vi "RT Main.vi"() -> ()   [LabVIEW 2015]
uses:
  <vilib>/robotics/Navigation/shared/WorldMap/DirectedGraphWorldMap/NI_Robotics_DirectedGraphWorldMap.lvclass
  NI-ARC 2017/NI ARC 2016/Types/Status.ctl
  Types/Mode.ctl
  <vilib>/myRIO/Instrument Drivers/Onboard IO/DIO/typedefs/DIO Reference.ctl
  <vilib>/myRIO/Common/Instrument Driver Framework/Utilities/typedefs/myRIO Generic Hardware Reference.ctl
  <vilib>/myRIO/Common/Instrument Driver Framework/Utilities/typedefs/Hardware Version Enum.ctl
  <vilib>/myRIO/Common/Instrument Driver Framework/Utilities/typedefs/myRIO v1.0 Reference.ctl
  <vilib>/myRIO/Common/Instrument Driver Framework/Utilities/typedefs/Generic FPGA Reference.ctl
  <vilib>/myRIO/Common/Instrument Driver Framework/myRIO v1.0/DIO/typedefs/DIO Channels List.ctl
  <vilib>/myRIO/Common/Instrument Driver Framework/myRIO v1.0/DIO/typedefs/DIO Channels Enum.ctl
  <vilib>/userdefined/High Color/nirio_resource_hc.ctl
  <vilib>/myRIO/Common/Instrument Driver Framework/Utilities/vis/Is FPGA Ref Available.vi
  <vilib>/myRIO/Common/Instrument Driver Framework/myRIO v1.0/DIO/vis/myRIO v1.1 Open DIO.vi
  <vilib>/myRIO/Instrument Drivers/Onboard IO/DIO/vis/Read.vi
  <vilib>/myRIO/Instrument Drivers/Onboard IO/DIO/vis/Write.vi
  <vilib>/myRIO/Common/Instrument Driver Framework/Utilities/vis/Validate Channels.vi
  <vilib>/myRIO/Common/Instrument Driver Framework/myRIO v1.0/DIO/vis/myRIO v1.0 Reserve DIO.vi
  <vilib>/myRIO/Common/Instrument Driver Framework/myRIO v1.0/Resource Manager/vis/myRIO v1.0 Reserve Channel List.vi
  <vilib>/myRIO/Common/Instrument Driver Framework/myRIO v1.0/DIO/vis/myRIO v1.0 Build MUX Configuration DIO.vi
  <vilib>/myRIO/Common/Instrument Driver Framework/myRIO v1.0/Resource Manager/vis/myRIO v1.0 Reserve Channel.vi
  <vilib>/myRIO/Common/Instrument Driver Framework/myRIO v1.0/Resource Manager/vis/myRIO v1.0 Unreserve Channel.vi
  <vilib>/myRIO/Common/Instrument Driver Framework/myRIO v1.0/Resource Manager/vis/myRIO v1.0 Create Configuration List.vi
  <vilib>/myRIO/Common/Instrument Driver Framework/myRIO v1.0/Resource Manager/vis/myRIO v1.0 Build Mutex Name.vi
  <vilib>/Utility/tcp.llb/UDP Multicast Read-Only Open.vi
  <vilib>/FPGAPlugInAG/myRIO-1900/niLvFpga_Open_myRIO-1900.vi
  <vilib>/rvi/interface/common/dynamic/niFpgaDynamicAddResources.vi
  <vilib>/myRIO/Common/Instrument Driver Framework/Utilities/vis/FPGA Ref Manager.vi
  <vilib>/Utility/error.llb/Error Cluster From Error Code.vi
  <vilib>/myRIO/Common/Instrument Driver Framework/Utilities/vis/Ref Counter.vi
  <vilib>/Utility/VariantDataType/GetNumericInfo.vi
  <vilib>/myRIO/Common/Instrument Driver Framework/myRIO v1.0/myRIO v1.1 Open.vi
  <vilib>/myRIO/Common/Instrument Driver Framework/Utilities/vis/IO Manager.vi
  <vilib>/myRIO/Common/Instrument Driver Framework/Utilities/vis/Configuration Manager.vi
  <vilib>/myRIO/Common/Instrument Driver Framework/myRIO v1.0/Resource Manager/vis/myRIO v1.0 Configure IO.vi
  <vilib>/myRIO/Common/Instrument Driver Framework/myRIO v1.0/myRIO v1.0 Close.vi
  <vilib>/myRIO/Common/Instrument Driver Framework/myRIO v1.0/DIO/vis/myRIO v1.0 Read DIO.vi
  <vilib>/myRIO/Common/Instrument Driver Framework/myRIO v1.0/DIO/vis/myRIO v1.0 Write DIO.vi
  <vilib>/FPGAPlugInAG/Dynamic/niLvFpga_Close_Dynamic.vi
  <vilib>/rvi/interface/nirviOpenFPGA/nirviOpenFPGA.xnode
  FPGA Bitfiles/NIARC2017_FPGATarget_FPGAMainDefault_FCosad5cmWo.lvbitx
  <vilib>/myRIO/Express VI/Onboard IO/DI/DI Express VI.xnode
  <vilib>/myRIO/Instrument Drivers/Onboard IO/DIO/vis/myRIO DIO Open.xnode
  <vilib>/myRIO/Express VI/Onboard IO/DO/DO Express VI.xnode
  <vilib>/rvi/interface/nirviCloseFPGA/nirviCloseFPGA.xnode
  <instrlib>/Hokuyo URG Series/HAIOL/Hokuyo URG Series.lvclass
  <vilib>/myRIO/Instrument Drivers/Utilities/Utilities.lvlib
  <instrlib>/Hokuyo URG Series/HAIOL/VISA/Hokuyo URG Series VISA.lvclass
  <vilib>/myRIO/Instrument Drivers/Onboard IO/DIO/DIO.lvlib
panel:
  in  "LidarDetection":bool
  out "x*y":dbl
  out "Next":T1
  out "wifiClosures":bool[](array[boolean])
  in  "MovingRobot":bool
  in  "Mode":T2
  in  "Status":T3
  out "Closures":bool[](array[boolean])
  out "closeLidar":cluster{dbl, dbl}[](array[cluster])
  out "Returning":bool=TRUE
  out "Last":string
  out "Wifi String":string
  out "error out":errorcluster
  out "Path":cluster{"name":string, "coordinates":dbl[]}[](array[cluster])
  out "Vertical Closures":bool[](array[boolean])
  in  "6":bool
  in  "5":bool
  in  "8":bool
  in  "7":bool
  in  "4":bool
  in  "3":bool
  in  "2":bool
  in  "1":bool
  out "No Valid Path":bool
  out "Horizontal Closures":bool[](array[boolean])
  in  "I":bool
  in  "H":bool
  in  "G":bool
  in  "F":bool
  in  "E":bool
  in  "D":bool
  in  "C":bool
  in  "B":bool
  in  "A":bool
  out "MapOut":refnum<data-value>
  out "Zones":T4(array[cluster])
  out "Obstacles":T4(array[cluster])
  out "Instruction":u32
  out "Start":T5
  in  "Finished":bool
  out "currentPath":T6
  out "Path":T7(array[cluster])=[{"pathSegment"={"Point 1"={"X"=250.0, "Y"=250.0}, "Point 2"={"X"=500.0, "Y"=250.0}}, "targetAngle"=0.0, "Speed"=1.0}, {"pathSegment"={"Point 1"={"X"=500.0, "Y"=250.0}, "Point 2"={"X"=300.0, "Y"=1500.0}}, "targetAngle"=90.0, "Speed"=1.0}, {"pathSegment"={"Point 1"={"X"=300.0, "Y"=1500.0}, "Point 2"={"X"=500.0, "Y"=3700.0}}, "targetAngle"=90.0, "Speed"=1.0}, {"pathSegment"={"Point 1"={"X"=500.0, "Y"=3700.0}, "Point 2"={"X"=3000.0, "Y"=3700.0}}, "targetAngle"=0.0, "Speed"=1.0}]
  out "plotPoints":cluster{dbl, dbl}[](array[cluster])
  out "Map":T8(plugin-control)
  out "lidarObstacles":T4(array[cluster])
  out "verticalCourse":cluster{"X":sgl, "Y":sgl}[](array[cluster])=[{"X"=-400.0, "Y"=600.0}, {"X"=-200.0, "Y"=600.0}, {"X"=0.0, "Y"=600.0}, {"X"=200.0, "Y"=600.0}, {"X"=400.0, "Y"=600.0}]
  out "hoizontalCourse":cluster{"X":sgl, "Y":sgl}[](array[cluster])=[{"X"=-400.0, "Y"=600.0}, {"X"=-200.0, "Y"=600.0}, {"X"=0.0, "Y"=600.0}, {"X"=200.0, "Y"=600.0}, {"X"=400.0, "Y"=600.0}]
  out "robotPosition":T5
  in  "Enable Motors":bool
  in  "Stop":bool
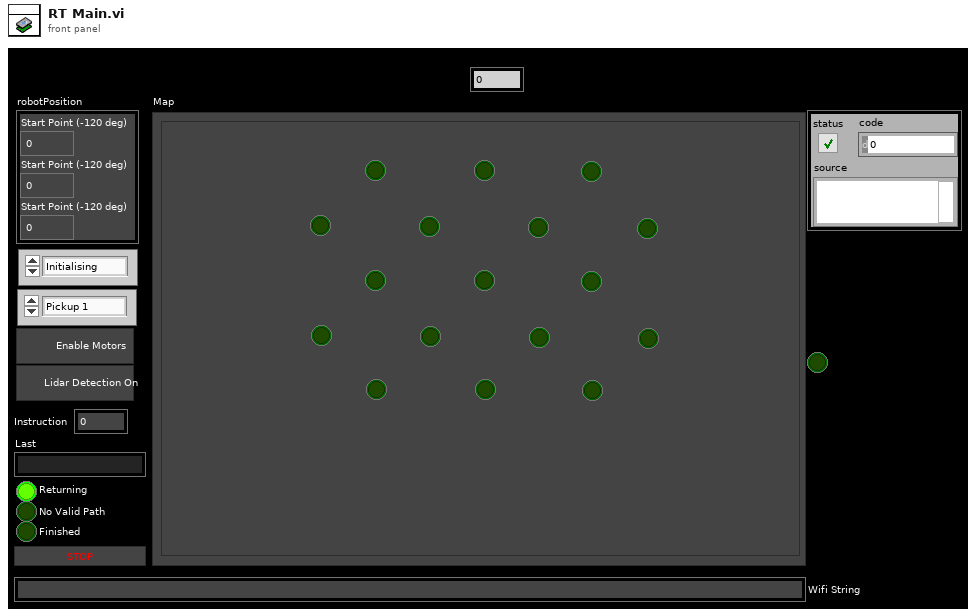
[diagram p1: front panel]
types:
  T1 = cluster{cluster{cluster{"Numeric":dbl, "Numeric":dbl}, cluster{"Numeric":dbl, "Numeric":dbl}}, "Ramp (V/s)":dbl, "Ramp (V/s)":dbl, bool}
  T2 = typedef "Mode.ctl" = enum16{"Pickup 1", "Pickup 2", "Moving Robot"}
  T3 = typedef "Status.ctl" = enum16{"Initialising", "Waiting", "Go"}
  T4 = cluster{"Point 1":cluster{"X":sgl, "Y":sgl}, "Point 2":cluster{"X":sgl, "Y":sgl}}[]
  T5 = cluster{"Start Point (-120 deg)":dbl, "Start Point (-120 deg)":dbl, "Start Point (-120 deg)":dbl}
  T6 = cluster{"pathSegment":cluster{"Point 1":cluster{"X":sgl, "Y":sgl}, "Point 2":cluster{"X":sgl, "Y":sgl}}, "targetAngle":dbl, "Speed":dbl}
  T7 = cluster{"pathSegment":cluster{"Point 1":cluster{"X":sgl, "Y":sgl}, "Point 2":cluster{"X":sgl, "Y":sgl}}, "targetAngle":dbl, "Speed":dbl}[]
  T8 = typedef "IMAQ Image.ctl" = refnum<image>
  T9 = typedef "DIO.lvlib/DIO Reference.ctl" = cluster{"myRIO Reference":T10, "DIO Channels List":T14}
  T10 = typedef "myRIO Generic Hardware Reference.ctl" = cluster{"myRIO Model":T11, "myRIO Hardware Reference":T12}
  T11 = typedef "Hardware Version Enum.ctl" = enum16{"Unknown", "myRIO-1900", "myRIO-1950", "roboRIO"}
  T12 = typedef "myRIO v1.0 Reference.ctl" = cluster{"Generic FPGA Reference":T13, "Allow multiple opens":bool}
  T13 = typedef "Generic FPGA Reference.ctl" = refnum<k20>
  T14 = typedef "DIO Channels List.ctl" = T15[]
  T15 = typedef "DIO Channels Enum.ctl" = enum16{"Not Connected", "C/DIO0", "C/DIO1", "C/DIO2", "C/DIO3", "C/DIO4", "C/DIO5", "C/DIO6", "C/DIO7", "A/DIO0", "A/DIO1", "A/DIO2", "A/DIO3", "A/DIO4", "A/DIO5", "A/DIO6", "A/DIO7", "A/DIO8", "A/DIO9", "A/DIO10", "A/DIO11", "A/DIO12", "A/DIO13", "A/DIO14", "A/DIO15", "B/DIO0", "B/DIO1", "B/DIO2", "B/DIO3", "B/DIO4", "B/DIO5", "B/DIO6", "B/DIO7", "B/DIO8", "B/DIO9", "B/DIO10", "B/DIO11", "B/DIO12", "B/DIO13", "B/DIO14", "B/DIO15", "LED0", "LED1", "LED2", "LED3", "Button0", "DIO/DIO0", "DIO/DIO1", "DIO/DIO2", "DIO/DIO3", "DIO/DIO4", "DIO/DIO5", "DIO/DIO6", "DIO/DIO7", "DIO/DIO8", "DIO/DIO9", "SPI/CS0", "SPI/CS1", "SPI/CS2", "SPI/CS3", "LED RADIO (Green)", "LED RADIO (Red)", "LED COMM (Green)", "LED COMM (Red)", "LED MODE (Green)", "LED MODE (Red)"}
  T16 = typedef "nirio_resource_hc.ctl" = tag
  T17 = cluster{cluster{cluster{"Numeric":dbl, "Numeric":dbl}, cluster{"Numeric":dbl, "Numeric":dbl}}, "Ramp (V/s)":dbl, "Ramp (V/s)":dbl}
  T18 = cluster{"Point 1":cluster{"X":sgl, "Y":sgl}, "Point 2":cluster{"X":sgl, "Y":sgl}}
  T19 = cluster{"x-Error":dbl, "y-Error":dbl, "Angle-Error (deg)":dbl}
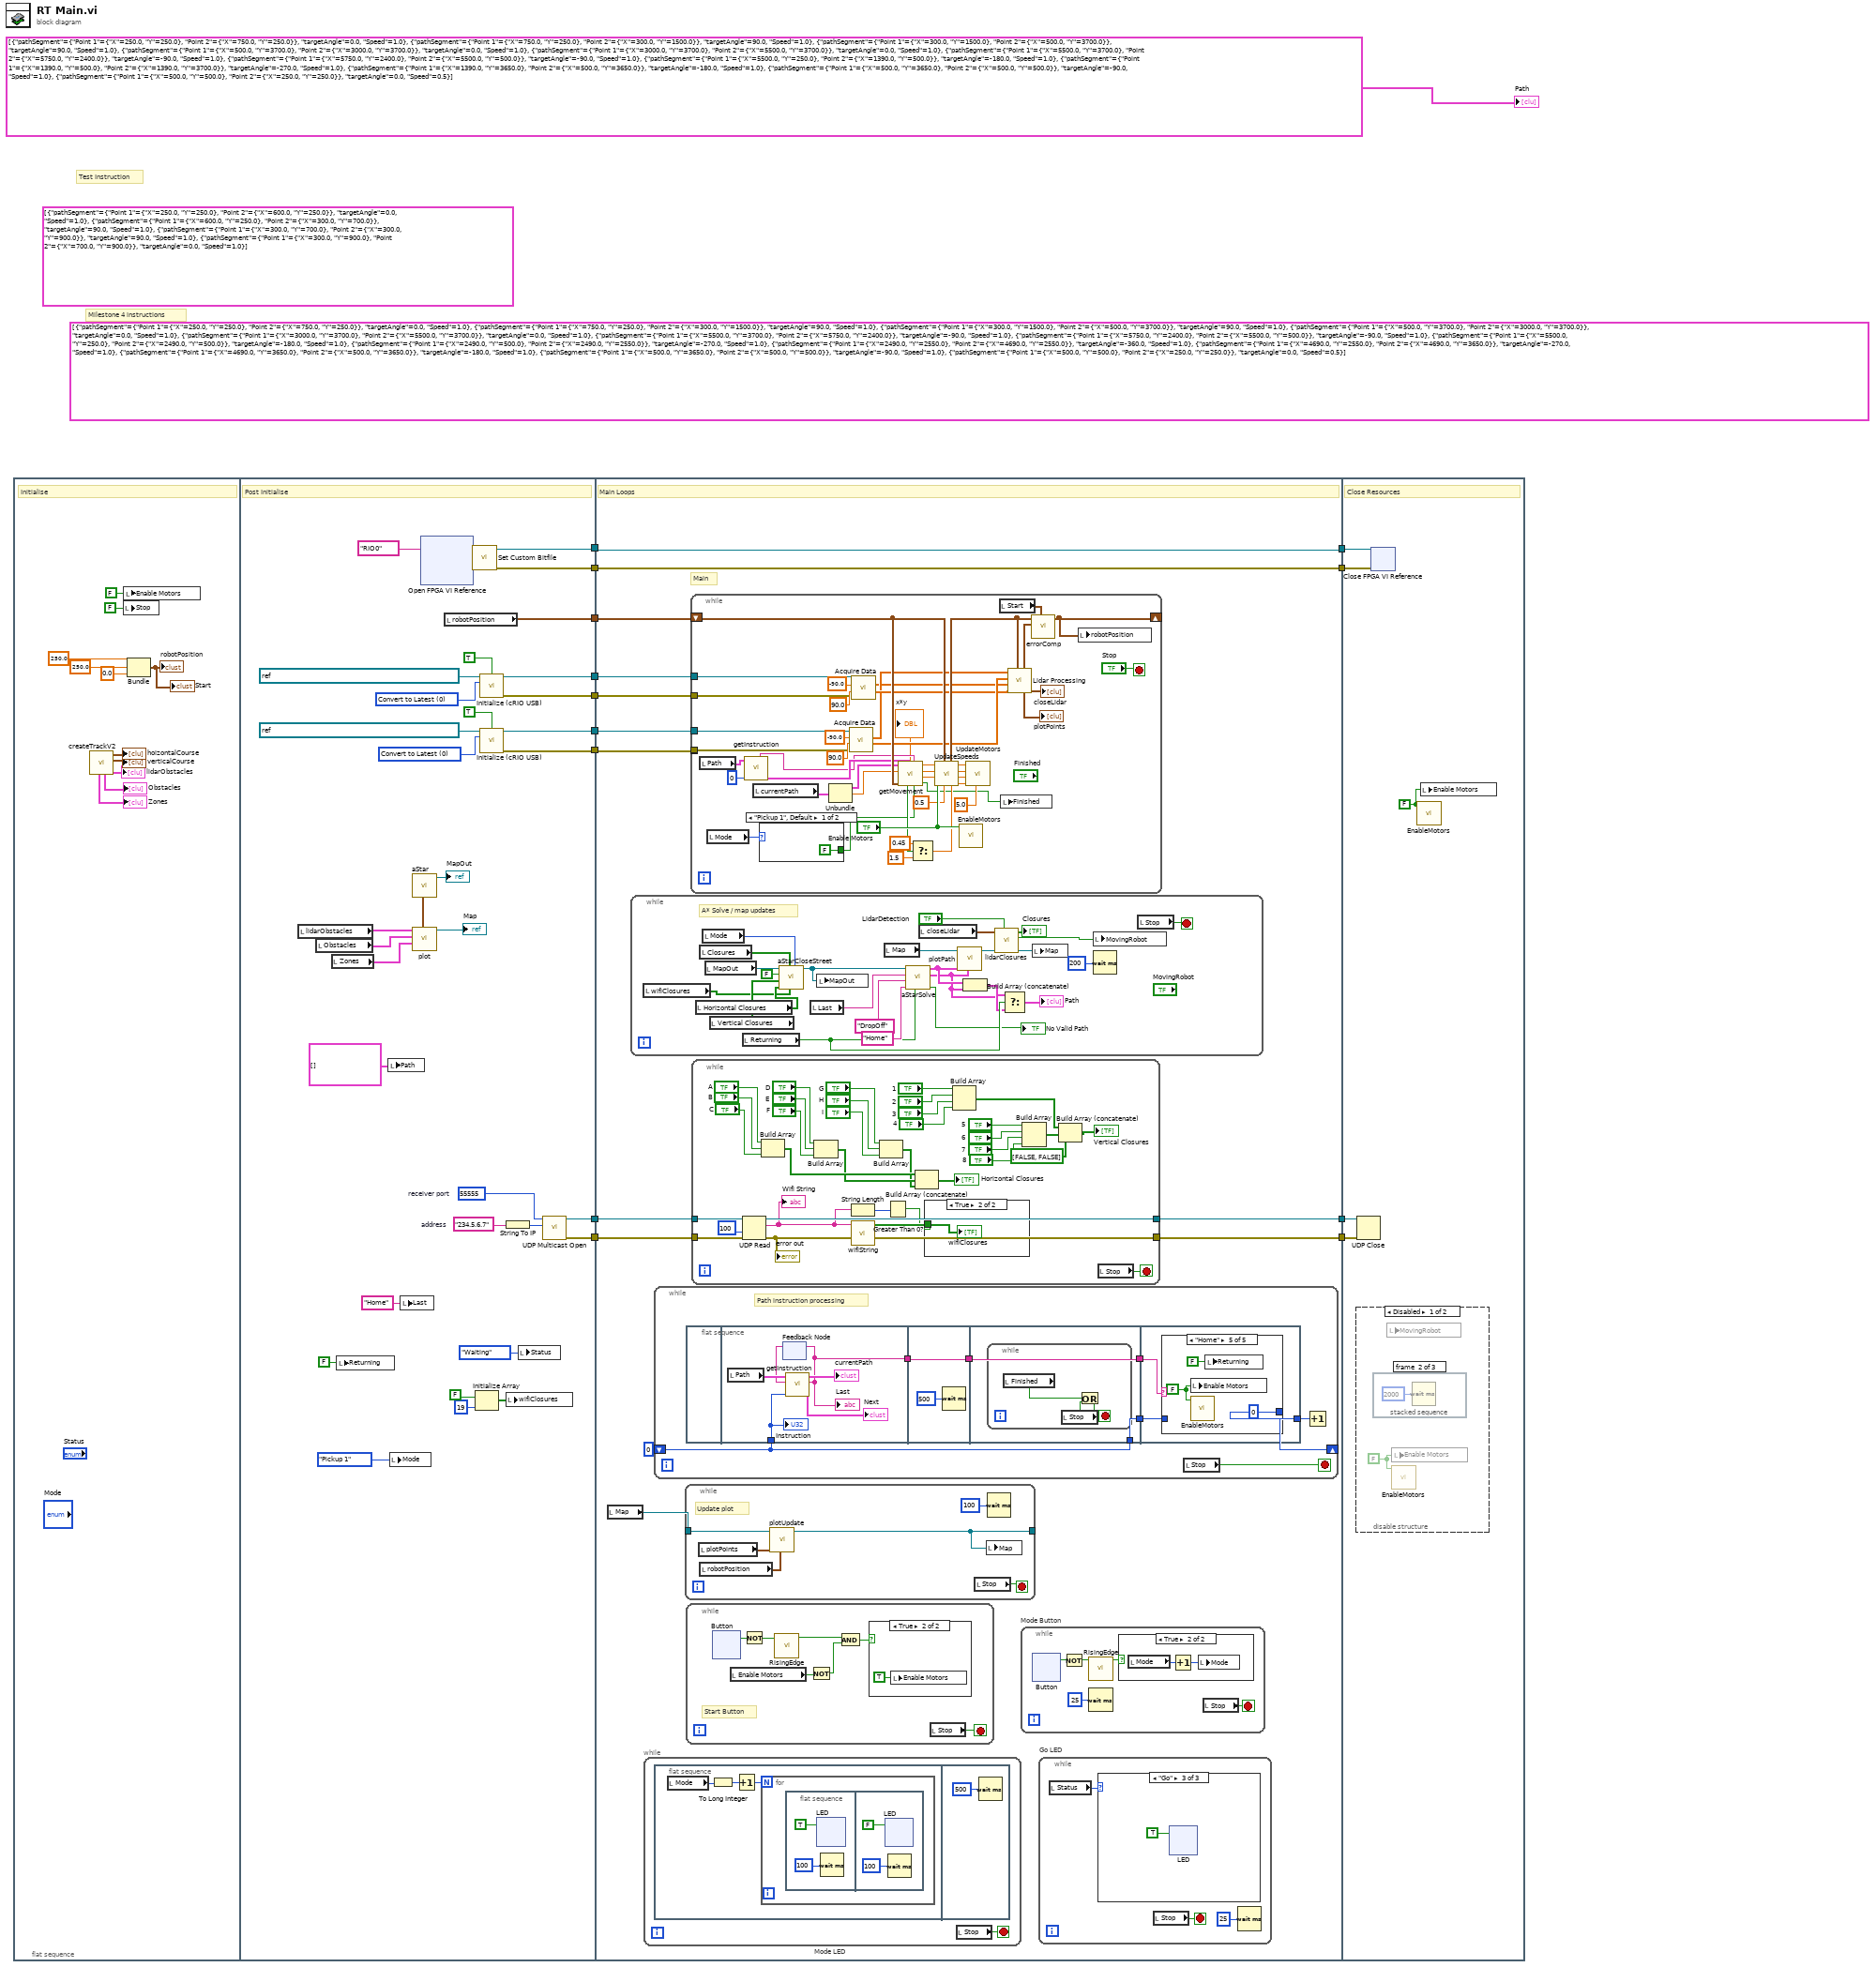
[diagram p0: block diagram]
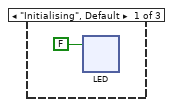
[diagram p3: hidden frame]
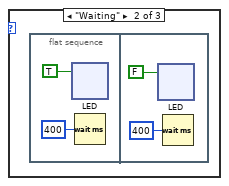
[diagram p4: hidden frame]
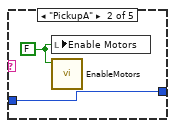
[diagram p8: hidden frame]
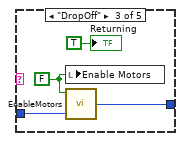
[diagram p9: hidden frame]
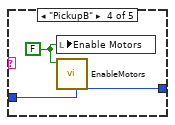
[diagram p10: hidden frame]
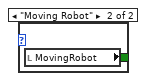
[diagram p11: hidden frame]
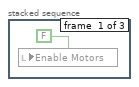
[diagram p12: hidden frame]
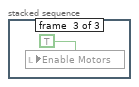
[diagram p13: hidden frame]
diagram:
  (unwired) T7 [{"pathSegment"={"Point 1"={"X"=250.0, "Y"=250.0}, "Point 2"={"X"=600.0, "Y"=250.0}}, "targetAngle"=0.0, "Speed"=1.0}, {"pathSegment"={"Point 1"={"X"=600.0, "Y"=250.0}, "Point 2"={"X"=300.0, "Y"=700.0}}, "targetAngle"=90.0, "Speed"=1.0}, {"pathSegment"={"Point 1"={"X"=300.0, "Y"=700.0}, "Point 2"={"X"=300.0, "Y"=900.0}}, "targetAngle"=90.0, "Speed"=1.0}, {"pathSegment"={"Point 1"={"X"=300.0, "Y"=900.0}, "Point 2"={"X"=700.0, "Y"=900.0}}, "targetAngle"=0.0, "Speed"=1.0}]
  (unwired) T7 [{"pathSegment"={"Point 1"={"X"=250.0, "Y"=250.0}, "Point 2"={"X"=750.0, "Y"=250.0}}, "targetAngle"=0.0, "Speed"=1.0}, {"pathSegment"={"Point 1"={"X"=750.0, "Y"=250.0}, "Point 2"={"X"=300.0, "Y"=1500.0}}, "targetAngle"=90.0, "Speed"=1.0}, {"pathSegment"={"Point 1"={"X"=300.0, "Y"=1500.0}, "Point 2"={"X"=500.0, "Y"=3700.0}}, "targetAngle"=90.0, "Speed"=1.0}, {"pathSegment"={"Point 1"={"X"=500.0, "Y"=3700.0}, "Point 2"={"X"=3000.0, "Y"=3700.0}}, "targetAngle"=0.0, "Speed"=1.0}, {"pathSegment"={"Point 1"={"X"=3000.0, "Y"=3700.0}, "Point 2"={"X"=5500.0, "Y"=3700.0}}, "targetAngle"=0.0, "Speed"=1.0}, {"pathSegment"={"Point 1"={"X"=5500.0, "Y"=3700.0}, "Point 2"={"X"=5750.0, "Y"=2400.0}}, "targetAngle"=-90.0, "Speed"=1.0}, {"pathSegment"={"Point 1"={"X"=5750.0, "Y"=2400.0}, "Point 2"={"X"=5500.0, "Y"=500.0}}, "targetAngle"=-90.0, "Speed"=1.0}, {"pathSegment"={"Point 1"={"X"=5500.0, "Y"=250.0}, "Point 2"={"X"=2490.0, "Y"=500.0}}, "targetAngle"=-180.0, "Speed"=1.0}, {"pathSegment"={"Point 1"={"X"=2490.0, "Y"=500.0}, "Point 2"={"X"=2490.0, "Y"=2550.0}}, "targetAngle"=-270.0, "Speed"=1.0}, {"pathSegment"={"Point 1"={"X"=2490.0, "Y"=2550.0}, "Point 2"={"X"=4690.0, "Y"=2550.0}}, "targetAngle"=-360.0, "Speed"=1.0}, {"pathSegment"={"Point 1"={"X"=4690.0, "Y"=2550.0}, "Point 2"={"X"=4690.0, "Y"=3650.0}}, "targetAngle"=-270.0, "Speed"=1.0}, {"pathSegment"={"Point 1"={"X"=4690.0, "Y"=3650.0}, "Point 2"={"X"=500.0, "Y"=3650.0}}, "targetAngle"=-180.0, "Speed"=1.0}, {"pathSegment"={"Point 1"={"X"=500.0, "Y"=3650.0}, "Point 2"={"X"=500.0, "Y"=500.0}}, "targetAngle"=-90.0, "Speed"=1.0}, {"pathSegment"={"Point 1"={"X"=500.0, "Y"=500.0}, "Point 2"={"X"=250.0, "Y"=250.0}}, "targetAngle"=0.0, "Speed"=0.5}]
  # "Milestone 4 instructions"
  # "Test Instruction"
  n1 = flat-sequence {
    tunnel: [w57] -> w14
    tunnel: [w56] -> w13
    tunnel: [w53] -> w12
    tunnel: [w52] -> w11
    tunnel: [w51] -> w8
    tunnel: [w42] -> w6
    tunnel: [w41] -> w5
    tunnel: [w35] -> w4
    tunnel: [w34] -> w3
    tunnel: w14 -> [w71]
    tunnel: w13 -> [w70]
    tunnel: w12 -> [w73]
    tunnel: w11 -> [w72]
    tunnel: [w71] -> w10
    tunnel: [w70] -> w9
    tunnel: w8 -> [w69]
    tunnel: w6 -> [w66]
    tunnel: w5 -> [w65]
    tunnel: w4 -> [w64]
    tunnel: w3 -> [w63]
    tunnel: [w62] -> w2
    tunnel: [w61] -> w1
    tunnel: w10 -> [w540]
    tunnel: w9 -> [w539]
    tunnel: w2 -> [w537]
    tunnel: w1 -> [w536]
    frame #0 {
      # "Initialise"
      n2 = call "createTrackV2.vi"() -> ("lidarObstacles"=→"lidarObstacles":T4, "verticalCourse"=→"verticalCourse":cluster{"X":sgl, "Y":sgl}[], "hoizontalCourse"=→"hoizontalCourse":cluster{"X":sgl, "Y":sgl}[], "obstacles"=→"Obstacles":T4, "Zones"=→"Zones":T4)  [unwired: 7 in]
      n3 = local write "Stop"(FALSE ("Stop")) -> ()
      n4 = local write "Enable Motors"(FALSE ("Enable Motors")) -> ()
      n5 = Bundle("Start Point (-120 deg)"=250.0, "Start Point (-120 deg)"=250.0, "Start Point (-120 deg)"=0.0) -> (→"robotPosition" →"Start":T5)  [unwired: 1 in]
    }
    frame #1 {
      w37 = u16 55555  # receiver port
      w38 = "234.5.6.7"  # address
      w44 = u32 0 items=["Convert to Latest", "SCIP 1.1", "SCIP 2.0"] ("Protocol (2: SCIP 2.0)")
      w54 = u32 0 items=["Convert to Latest", "SCIP 1.1", "SCIP 2.0"] ("Protocol (2: SCIP 2.0)")
      # "Post Initialise"
      n6 = local read "lidarObstacles"() -> (w50:T4)
      n7 = local read "Obstacles"() -> (w48:T4)
      n8 = local read "Zones"() -> (w47:T4)
      n9 = local write "Returning"(FALSE ("Returning")) -> ()
      n10 = local write "Path"(cluster{"name":string, "coordinates":dbl[]}[] [] ("Path")) -> ()
      n11 = local write "Mode"(Mode."Pickup 1" ("Mode")) -> ()
      n12 = local write "Last"("Home" ("Last")) -> ()
      n13 = call "aStar.vi"() -> ("MapOut"=→"MapOut":refnum<data-value>, "wayPoints"=w40:cluster{"Numeric":dbl, "Numeric":dbl}[])  [unwired: 10 in]
      n14 = call "plot.vi"("wayPoints"=w40, "Zones"=w47, "Obstacles"=w48, "Lidar"=w50) -> ("Image"=→"Map":T8)  [unwired: 7 in]
      n15 = xnode "Open FPGA VI Reference"("resource name"=tag "RIO0") -> ("FPGA VI Reference Out"=w58:refnum<k20>, "error out"=w59:errorcluster)  [unwired: 1 in]
      n16 = local read "robotPosition"() -> (w51:T5)
      n17 = call <vilib>:"Set Custom Bitfile.vi"("error in (no error)"=w59, "Custom FPGA Reference In"=w58) -> ("error out"=w56:errorcluster, "Custom FPGA Reference Out"=w57:refnum<k20>)  [unwired: 8 in]
      n18 = Initialize Array(FALSE ("Returning"), 19 ("dimension size")) -> (w28:bool[])
      n19 = call <instrlib>:"Initialize (cRIO USB).vi"("VISA resource name"=refnum<visa-resource-name> "USB0::0x15D1::0x0000::NI-VISA-1003::1::RAW", "Reset? (F: No)"=TRUE, "Protocol (2: SCIP 2.0)"=w54) -> ("Hokuyo URG Series out"=w53:refnum<class "Hokuyo URG Series.lvclass">, "error out"=w52:errorcluster)  [unwired: 11 in]
      n20 = call <instrlib>:"Initialize (cRIO USB).vi"("VISA resource name"=refnum<visa-resource-name> "USB0::0x15D1::0x0000::NI-VISA-1004::1::RAW", "Reset? (F: No)"=TRUE, "Protocol (2: SCIP 2.0)"=w44) -> ("Hokuyo URG Series out"=w42:refnum<class "Hokuyo URG Series.lvclass">, "error out"=w41:errorcluster)  [unwired: 11 in]
      n21 = String To IP(1:w38) -> (0:w36:u32)
      n22 = local write "wifiClosures"(w28) -> ()
      n23 = local write "Status"(Status."Waiting" ("Status")) -> ()
      n24 = call-poly <vilib>:"UDP Multicast Open.vi"("multicast addr"=w36, "port"=w37) -> ("error out"=w34:errorcluster, "connection ID"=w35:refnum<k16>)  [unwired: 7 in, 1 out]
    }
    frame #2 {
      # "Main"
      # "Main Loops"
      n25 = local read "Map"() -> (w68:T8)
      n26 = while {
        stop <- w385 stop-if-true
        # "A* Solve / map updates"
        n27 = local read "wifiClosures"() -> (w382:bool[])
        n28 = local read "Horizontal Closures"() -> (w401:bool[])
        n29 = local read "Closures"() -> (w388:bool[])
        n30 = local read "Mode"() -> (w387:T2)
        n31 = local read "MapOut"() -> (w403:refnum<data-value>)
        n32 = local read "Vertical Closures"() -> (w383:bool[])
        n33 = local read "Returning"() -> (w396:bool)
        n34 = call "aStarCloseStreet.vi"("Mode"=w387, "wifiClosures"=w382, "Lidar Closures"=w388, "Horizontal Closures"=w401, "Vertical Closures"=w383, "MovingRobot"=FALSE, "MapIn"=w403) -> ("MapOut"=w402:refnum<data-value>)  [unwired: 4 in]
        n35 = local read "Last"() -> (w397:string)
        n36 = local write "MapOut"(w402) -> ()
        n37 = local read "Map"() -> (w405:T8)
        n38 = call "aStarSolve.vi"("Returning"=w396, "Home"="Home", "Goal"="DropOff" ("Start"), "Last"=w397, "MapOut"=w402) -> ("no valid path exists"=→"No Valid Path":bool, "returnNodes"=w394:cluster{"name":string, "coordinates":dbl[]}[], "nodes"=w400:cluster{"name":string, "coordinates":dbl[]}[])  [unwired: 4 in]
        n39 = local read "closeLidar"() -> (w390:cluster{dbl, dbl}[])
        n40 = call "plotPath.vi"("ReturnNodes"=w394, "nodes"=w400, "Image"=w405) -> ("imageOut"=w392:T8)  [unwired: 8 in]
        n41 = Build Array (concatenate)(w400, w394) -> (w395:cluster{"name":string, "coordinates":dbl[]}[])
        n42 = call "lidarClosures.vi"("lidarClosureOn"="LidarDetection", "Image"=w392, "plotPoints"=w390) -> ("Image Out"=w391:T8, "MovingRobot"=w384:bool, "Closures"=→"Closures":bool[])  [unwired: 6 in]
        n43 = Select(t=w394, s=w396, f=w395) -> (s? t:f=→"Path":cluster{"name":string, "coordinates":dbl[]}[])
        n44 = local write "Map"(w391) -> ()
        n45 = local write "MovingRobot"(w384) -> ()
        n46 = Wait (ms)(milliseconds to wait=u32 200) -> ()  [unwired: 1 out]
        n47 = local read "Stop"() -> (w385:bool)
      }
      n48 = while "Mode LED" {
        stop <- w116 stop-if-true
        n49 = flat-sequence {
          frame #0 {
            n50 = local read "Mode"() -> (w117:T2)
            n51 = To Long Integer(number=w117) -> (32bit integer=w118:i32)
            n52 = Increment(x=w118) -> (x+1=w119:i32)
            n53 = for {
              N: w119 -> [_]
              n54 = flat-sequence {
                frame #0 {
                  n55 = xnode "LED"("A/DIO2 (Pin 15)"=TRUE ("A/DIO4 (Pin 19)")) -> ()  [unwired: 1 in, 1 out]
                  n56 = Wait (ms)(milliseconds to wait=u32 100) -> ()  [unwired: 1 out]
                }
                frame #1 {
                  n57 = xnode "LED"("A/DIO2 (Pin 15)"=FALSE ("A/DIO4 (Pin 19)")) -> ()  [unwired: 1 in, 1 out]
                  n58 = Wait (ms)(milliseconds to wait=u32 100) -> ()  [unwired: 1 out]
                }
              }
            }
          }
          frame #1 {
            n59 = Wait (ms)(milliseconds to wait=u32 500) -> ()  [unwired: 1 out]
          }
        }
        n60 = local read "Stop"() -> (w116:bool)
      }
      n61 = while {
        shift-right: [w449] -> _
        shift-left: u32 0 ("millisecond multiple") -> [w455]
        stop <- w454 stop-if-true
        # "Path instruction processing"
        n62 = flat-sequence {
          tunnel: w455 -> [w460]
          tunnel: [w458] -> w452
          tunnel: w452 -> [w462]
          tunnel: [w462] -> w451
          tunnel: w455 -> [w465]
          tunnel: [w465] -> w453
          tunnel: w451 -> [w464]
          tunnel: [w464] -> w450
          tunnel: w453 -> [w470]
          tunnel: [w471] -> w449
          tunnel: w450 -> [w469]
          frame #0 {
          }
          frame #1 {
            n63 = local read "Path"() -> (w461:cluster{"name":string, "coordinates":dbl[]}[])
            n64 = feedback #1() -> (w457:string)  [unwired: 1 in]
            n65 = call "getInstruction.vi"("index"=w460, "PrevLast"=w457, "Path"=w461) -> ("Next"=→"Next":T1, "Node"=w458:string, "CurrentPath"=→"currentPath":T17)  [unwired: 5 in, 1 out]
            "Last" <- w458
            n66 = feedback-in #1(w458) -> ()
            "Instruction" <- w460
          }
          frame #2 {
            n67 = Wait (ms)(milliseconds to wait=u32 500) -> ()  [unwired: 1 out]
          }
          frame #3 {
            n68 = while {
              stop <- w468 stop-if-true
              n69 = local read "Finished"() -> (w466:bool)
              n70 = local read "Stop"() -> (w467:bool)
              n71 = Or(x=w466, y=w467) -> (x .or. y?=w468:bool)
            }
          }
          frame #4 {
            n72 = case shown="\"Home\"" w469 {
              tunnel: w470 -> [w472 w474 w477 w479 _]
              tunnel: [w472 w474 w477 w479 u32 0 ("millisecond multiple")] -> w471
              frame "0", Default {
              }
              frame "PickupA" {
                w473 = FALSE ("Enabled?")
                n73 = local write "Enable Motors"(w473) -> ()
                n74 = call "EnableMotors.vi"("Enabled?"=w473) -> ()  [unwired: 11 in]
              }
              frame "DropOff" {
                w475 = FALSE ("Enabled?")
                n75 = local write "Enable Motors"(w475) -> ()
                n76 = call "EnableMotors.vi"("Enabled?"=w475) -> ()  [unwired: 11 in]
                "Returning" <- TRUE ("Boolean")
              }
              frame "PickupB" {
                w478 = FALSE ("Enabled?")
                n77 = local write "Enable Motors"(w478) -> ()
                n78 = call "EnableMotors.vi"("Enabled?"=w478) -> ()  [unwired: 11 in]
              }
              frame "Home" {
                w481 = FALSE ("Enabled?")
                n79 = local write "Enable Motors"(w481) -> ()
                n80 = call "EnableMotors.vi"("Enabled?"=w481) -> ()  [unwired: 11 in]
                n81 = local write "Returning"(FALSE ("Returning")) -> ()
              }
            }
          }
        }
        n82 = local read "Stop"() -> (w454:bool)
        n83 = Increment(x=w449) -> ()  [unwired: 1 out]
      }
      n84 = while {
        tunnel: w68 -> [w486]
        tunnel: [w483] -> _
        stop <- w488 stop-if-true
        # "Update plot"
        n85 = local read "plotPoints"() -> (w485:cluster{dbl, dbl}[])
        n86 = local read "robotPosition"() -> (w484:T5)
        n87 = call "plotUpdate.vi"("robotPosition"=w484, "plotPoints"=w485, "Image"=w486) -> ("imageOut"=w483:T8)  [unwired: 8 in]
        n88 = local read "Stop"() -> (w488:bool)
        n89 = local write "Map"(w483) -> ()
        n90 = Wait (ms)(milliseconds to wait=u32 100) -> ()  [unwired: 1 out]
      }
      n91 = while {
        stop <- w412 stop-if-true
        # "Start Button"
        n92 = xnode "Button"() -> ("A/DIO5 (Pin 21)"=w406:bool)  [unwired: 1 in, 1 out]
        n93 = local read "Enable Motors"() -> (w408:bool)
        n94 = Not(x=w406) -> (.not. x?=w411:bool)
        n95 = call "RisingEdge.vi"("Input"=w411) -> ("Rising?"=w410:bool)  [unwired: 10 in]
        n96 = Not(x=w408) -> (.not. x?=w409:bool)
        n97 = And(x=w410, y=w409) -> (x .and. y?=w407:bool)
        n98 = case shown="True" w407 {
          frame False {
          }
          frame True {
            n99 = local write "Enable Motors"(TRUE ("Enable Motors")) -> ()
          }
        }
        n100 = local read "Stop"() -> (w412:bool)
      }
      n101 = while {
        tunnel: w73 -> [w530]
        tunnel: w72 -> [w529]
        shift-right: [w515] -> _
        shift-left: w69 -> [w514]
        tunnel: w66 -> [w503]
        tunnel: [w502] -> _
        tunnel: w65 -> [w502]
        stop <- "Stop" stop-if-true
        n102 = local read "Path"() -> (w493:cluster{"name":string, "coordinates":dbl[]}[])
        n103 = local read "Mode"() -> (w495:T2)
        n104 = call "getInstruction.vi"("index"=0, "Path"=w493) -> ("Next"=w491:T1, "Last"=w490:string)  [unwired: 6 in, 2 out]
        n105 = local read "currentPath"() -> (w513:T6)
        n106 = case shown="\"Pickup 1\", Default" w495 {
          tunnel: [FALSE ("MovingRobot") w535] -> w494
          frame "Pickup 1", Default {
          }
          frame "Moving Robot" {
            n107 = local read "MovingRobot"() -> (w535:bool)
          }
        }
        n108 = Unbundle(w513) -> ("pathSegment"=w512:T18, "targetAngle"=w511:dbl)  [unwired: 1 out]
        n109 = call-dynamic "Acquire Data.vi"("error in (no error)"=w502, "End Point (120 deg)"=90.0, "Start Point (-120 deg)"=-90.0, "Hokuyo URG Series in"=w503) -> ("Direction"=w501:dbl[], "Magnitude"=w497:dbl[])  [unwired: 4 in, 2 out]
        n110 = call-dynamic "Acquire Data.vi"("error in (no error)"=w529, "End Point (120 deg)"=90.0, "Start Point (-120 deg)"=-90.0, "Hokuyo URG Series in"=w530) -> ("Direction"=w498:dbl[], "Magnitude"=w496:dbl[])  [unwired: 4 in, 2 out]
        n111 = call "getMovement.vi"("NoValidPath"=w494, "Last"=w490, "Next"=w491, "robotPosition"=w514, "targetAngle"=w511, "pathSegment"=w512) -> ("finshed"=w500:bool, "Rotational Velocity"=w521:dbl, "Left"=w522:dbl, "Forwards"=w523:dbl, "Slowdown"=w508:bool, "x*y"=→"x*y":dbl)
        n112 = Select(t=0.45, s=w508, f=1.5 ("SpeedMutiplier")) -> (s? t:f=w506:dbl)
        n113 = call "UpdateSpeeds.vi"("SpeedMutiplier"=w506, "Ramp (V/s)"=0.5, "robotPositionIn"=w514, "Enabled"="Enable Motors", "Rotation (V)"=w521, "Left/Right (V)"=w522, "Forwards/Back (V)"=w523) -> ("M4 (V)"=w524:dbl, "M3 (V)"=w525:dbl, "M2 (V)"=w526:dbl, "M1 (V)"=w527:dbl, "robotPositionOut"=w516:T5)
        n114 = call "EnableMotors.vi"("Enabled?"="Enable Motors") -> ()  [unwired: 11 in]
        n115 = call "UpdateMotors.vi"("Ramp (V/s)"=5.0, "M4 (V)"=w524, "M3 (V)"=w525, "M2 (V)"=w526, "M1 (V)"=w527) -> ()  [unwired: 7 in]
        n116 = local read "Start"() -> (w510:T5)
        n117 = local write "Finished"(w500) -> ()
        n118 = call "Lidar Processing.vi"("robotPosition"=w516, "Direction 2"=w498, "Magnitude 2"=w496, "Direction"=w501, "Magnitude"=w497) -> ("closeLidar"=→"closeLidar":cluster{dbl, dbl}[], "plotPoints"=→"plotPoints":cluster{dbl, dbl}[], "Error"=w517:T19)  [unwired: 3 in, 1 out]
        n119 = call "errorComp.vi"("Start"=w510, "Error"=w517, "Position"=w516) -> ("Compesated Position"=w515:T5)  [unwired: 8 in]
        n120 = local write "robotPosition"(w515) -> ()
      }
      n121 = while {
        tunnel: w64 -> [w352]
        tunnel: w63 -> [w351]
        tunnel: [w350] -> w62
        tunnel: [w349] -> w61
        stop <- w354 stop-if-true
        n122 = UDP Read(connection ID=w352, timeout ms (25000)=100, 8:w351) -> (data out=w347:string, error out=w349:errorcluster, 3:w350:refnum<k16>)  [unwired: 3 out]
        "error out" <- w349
        "Wifi String" <- w347
        n123 = Build Array("A", "B", "C") -> (w358:bool[])
        n124 = Build Array("D", "E", "F") -> (w357:bool[])
        n125 = String Length(string=w347) -> (length=w346:i32)
        n126 = call "wifiString.vi"("wifiString"=w347) -> ("Closures"=w345:bool[])  [unwired: 10 in]
        n127 = Build Array("G", "H", "I") -> (w356:bool[])
        n128 = Greater Than 0?(x=w346) -> (x > 0?=w344:bool)
        n129 = Build Array (concatenate)(w358, w357, w356) -> (→"Horizontal Closures":bool[])
        n130 = case shown="True" w344 {
          tunnel: w345 -> [_ w379]
          frame False {
          }
          frame True {
            "wifiClosures" <- w379
          }
        }
        n131 = Build Array("1", "2", "3", "4") -> (w377:bool[])
        n132 = Build Array("5", "6", "7", "8") -> (w376:bool[])
        n133 = Build Array (concatenate)(w377, w376, bool[] [FALSE, FALSE] ("array")) -> (→"Vertical Closures":bool[])
        n134 = local read "Stop"() -> (w354:bool)
      }
      n135 = while "Mode Button" {
        stop <- w78 stop-if-true
        n136 = xnode "Button"() -> ("A/DIO3 (Pin 17)"=w76:bool)  [unwired: 1 in, 1 out]
        n137 = Not(x=w76) -> (.not. x?=w75:bool)
        n138 = call "RisingEdge.vi"("Input"=w75) -> ("Rising?"=w74:bool)  [unwired: 10 in]
        n139 = Wait (ms)(milliseconds to wait=u32 25) -> ()  [unwired: 1 out]
        n140 = case shown="True" w74 {
          frame False {
          }
          frame True {
            n141 = local read "Mode"() -> (w80:T2)
            n142 = Increment(x=w80) -> (x+1=w79:T2)
            n143 = local write "Mode"(w79) -> ()
          }
        }
        n144 = local read "Stop"() -> (w78:bool)
      }
      n145 = while "Go LED" {
        stop <- w196 stop-if-true
        n146 = local read "Status"() -> (w197:T3)
        n147 = case shown="\"Go\"" w197 {
          frame "Initialising", Default {
            n148 = xnode "LED"("A/DIO4 (Pin 19)"=FALSE) -> ()  [unwired: 1 in, 1 out]
          }
          frame "Waiting" {
            n149 = flat-sequence {
              frame #0 {
                n150 = xnode "LED"("A/DIO4 (Pin 19)"=TRUE) -> ()  [unwired: 1 in, 1 out]
                n151 = Wait (ms)(milliseconds to wait=u32 400) -> ()  [unwired: 1 out]
              }
              frame #1 {
                n152 = xnode "LED"("A/DIO4 (Pin 19)"=FALSE) -> ()  [unwired: 1 in, 1 out]
                n153 = Wait (ms)(milliseconds to wait=u32 400) -> ()  [unwired: 1 out]
              }
            }
          }
          frame "Go" {
            n154 = xnode "LED"("A/DIO4 (Pin 19)"=TRUE) -> ()  [unwired: 1 in, 1 out]
          }
        }
        n155 = local read "Stop"() -> (w196:bool)
        n156 = Wait (ms)(milliseconds to wait=u32 25) -> ()  [unwired: 1 out]
      }
    }
    frame #3 {
      w538 = FALSE ("Enabled?")
      # "Close Resources"
      n157 = disable-structure shown="Disabled" {
        frame Disabled {
          w541 = FALSE ("Enabled?")
          n158 = stacked-sequence {
            frame #0 {
              n159 = local write "Enable Motors"(FALSE ("Enabled?")) -> ()
            }
            frame #1 {
              n160 = Wait (ms)(milliseconds to wait=u32 2000) -> ()  [unwired: 1 out]
            }
            frame #2 {
              n161 = local write "Enable Motors"(TRUE ("Enabled?")) -> ()
            }
          }
          n162 = local read "MovingRobot"() -> ()  [unwired: 1 in]
          n163 = local write "Enable Motors"(w541) -> ()
          n164 = call "EnableMotors.vi"("Enabled?"=w541) -> ()  [unwired: 11 in]
        }
        frame Enabled {
        }
      }
      n165 = UDP Close(connection ID=w537, 8:w536) -> ()  [unwired: 2 out]
      n166 = xnode "Close FPGA VI Reference"("FPGA VI Reference In"=w540, "error in"=w539) -> ()  [unwired: 1 out]
      n167 = call "EnableMotors.vi"("Enabled?"=w538) -> ()  [unwired: 11 in]
      n168 = local write "Enable Motors"(w538) -> ()
    }
  }
  "Path" <- T7 [{"pathSegment"={"Point 1"={"X"=250.0, "Y"=250.0}, "Point 2"={"X"=750.0, "Y"=250.0}}, "targetAngle"=0.0, "Speed"=1.0}, {"pathSegment"={"Point 1"={"X"=750.0, "Y"=250.0}, "Point 2"={"X"=300.0, "Y"=1500.0}}, "targetAngle"=90.0, "Speed"=1.0}, {"pathSegment"={"Point 1"={"X"=300.0, "Y"=1500.0}, "Point 2"={"X"=500.0, "Y"=3700.0}}, "targetAngle"=90.0, "Speed"=1.0}, {"pathSegment"={"Point 1"={"X"=500.0, "Y"=3700.0}, "Point 2"={"X"=3000.0, "Y"=3700.0}}, "targetAngle"=0.0, "Speed"=1.0}, {"pathSegment"={"Point 1"={"X"=3000.0, "Y"=3700.0}, "Point 2"={"X"=5500.0, "Y"=3700.0}}, "targetAngle"=0.0, "Speed"=1.0}, {"pathSegment"={"Point 1"={"X"=5500.0, "Y"=3700.0}, "Point 2"={"X"=5750.0, "Y"=2400.0}}, "targetAngle"=-90.0, "Speed"=1.0}, {"pathSegment"={"Point 1"={"X"=5750.0, "Y"=2400.0}, "Point 2"={"X"=5500.0, "Y"=500.0}}, "targetAngle"=-90.0, "Speed"=1.0}, {"pathSegment"={"Point 1"={"X"=5500.0, "Y"=250.0}, "Point 2"={"X"=1390.0, "Y"=500.0}}, "targetAngle"=-180.0, "Speed"=1.0}, {"pathSegment"={"Point 1"={"X"=1390.0, "Y"=500.0}, "Point 2"={"X"=1390.0, "Y"=3700.0}}, "targetAngle"=-270.0, "Speed"=1.0}, {"pathSegment"={"Point 1"={"X"=1390.0, "Y"=3650.0}, "Point 2"={"X"=500.0, "Y"=3650.0}}, "targetAngle"=-180.0, "Speed"=1.0}, {"pathSegment"={"Point 1"={"X"=500.0, "Y"=3650.0}, "Point 2"={"X"=500.0, "Y"=500.0}}, "targetAngle"=-90.0, "Speed"=1.0}, {"pathSegment"={"Point 1"={"X"=500.0, "Y"=500.0}, "Point 2"={"X"=250.0, "Y"=250.0}}, "targetAngle"=0.0, "Speed"=0.5}]
